vi "Setup UI.vi"(8 "error in (no error)":errorcluster, 10 "Set UI to input? (F)":bool, 11 "multimeter reader in":refnum<class "multimeter reader.lvclass">) -> (0 "error out":errorcluster, 3 "multimeter reader out":refnum<class "multimeter reader.lvclass">)   [LabVIEW 2015, in "multimeter reader.lvclass"]
doc: "Setup UI constructs an object -- populates its member fields -- from a front panel the user can see. The VI should be as simple as possible so that a UI loop can poll it continuously for updates. \n\nThe VI is designed to be used as a subPanel within another VI. Wire true to \"Set UI to input\" only on the first call, just after inserting this VI into a subPanel, to populate its controls with the class's current values.\n\nSetup UI is distinct from the class constructor. Class constructors are not polymorphic, yet configure dialogs need to configure objects without knowing their type -- and polymorphism is the necessary solution. Thus, Setup UI is a polymorphic class constructor. This continously polled \"Setup UI\" concept is a kludge: a better idea would be an XControl, but those require a steeper learning curve."
uses:
  multimeter reader.lvclass
  multimeter reader.lvclass/multimeter reader.ctl
  Reader/Reader.lvclass
panel:
  in  "trigger mode set":u16(ring) items=["internal - continuous trigger", "external - rear panel trigger with delay", "external - bus trigger with delay", "external - rear panel trigger", "external - bus trigger"]
  in  "rate set":u16(ring) items=["slow", "medium", "fast"]
  in  "range set":u16(ring)=6 items=["autorange", "200mV, 200 ohms", "2V, 2 kohms", "20V, 20 kohms", "200V, 200 kohms", "1000Vdc, 700 Vac, 2 Mohms", "20 Mohms"]
  in  "function set":u16(ring) items=["volts DC", "volts AC", "2-wire k.ohms", "4-wire k.ohms", "mA DC", "mA AC"]
  # "Multimeter Control Setup"
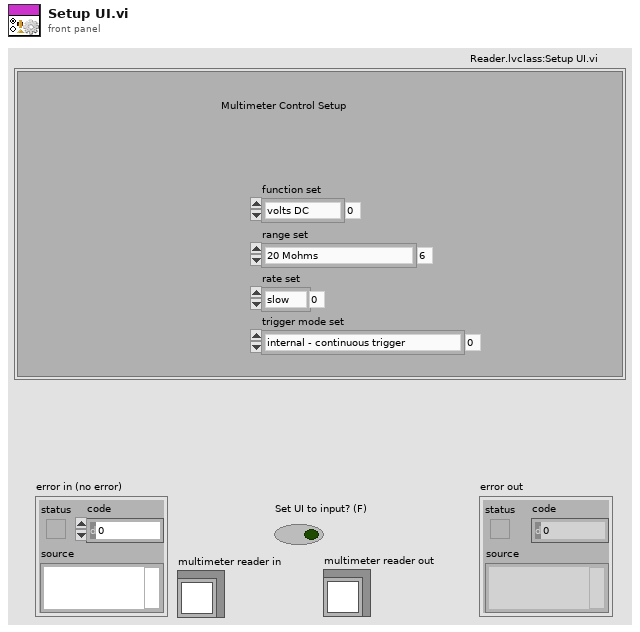
[diagram p1: front panel]
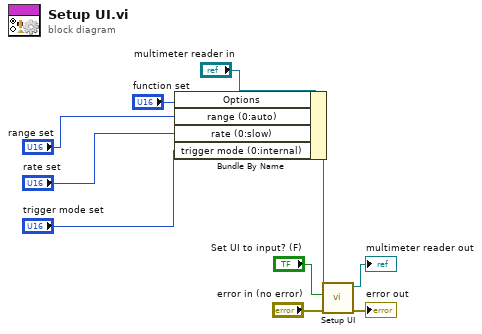
[diagram p0: block diagram]
diagram:
  n1 = Bundle By Name(cluster="multimeter reader in", "Options"="function set", "range (0:auto)"="range set", "rate (0:slow)"="rate set", "trigger mode (0:internal)"="trigger mode set") -> (w6:refnum<class "multimeter reader.lvclass">)
  n2 = call-parent "Setup UI.vi"("error in (no error)"="error in (no error)", "Set UI to input? (F)"="Set UI to input? (F)", "Reader in"=w6) -> ("error out"=→"error out":errorcluster, "Reader out"=→"multimeter reader out":refnum<class "multimeter reader.lvclass">)  [unwired: 7 in]
